vi "HEC28_PEMFC_UserInterface-Testing.vi"() -> ()   [LabVIEW 2020]
uses:
  <vilib>/MakerHub/LINX/Public/Peripherals/Digital/Digital Write 1 Chan.vi
  <vilib>/MakerHub/LINX/Public/Peripherals/Digital/Digital Write N Chans.vi
  <vilib>/MakerHub/LINX/Private/Local IO/LinxDigitalWrite.vi
  <vilib>/MakerHub/LINX/Public/Utilities/Check Channel.vi
  <vilib>/MakerHub/LINX/Public/Utilities/Open Serial.vi
  <instrlib>/NI RMX-400x Loads/Public/Data/Fetch All Measurements (Current).vi
  <instrlib>/NI RMX-400x Loads/Public/Data/Fetch All Measurements (Power).vi
  <instrlib>/NI RMX-400x Loads/Public/Data/Fetch All Measurements (Voltage).vi
  <vilib>/MakerHub/LINX/Private/Utilties/Generate Error.vi
  <vilib>/MakerHub/LINX/LMH-LINX.lvlib
  <instrlib>/NI RMX-400x Loads/NI RMX-400x Loads.lvlib
panel:
  in  "Set Purge Time":dbl=30.0 format="%#_13g"
  in  "Flowrate(SLPM)":dbl=1.5
  out "Power Waveform":dbl[][](graph)
  out "Voltage Waveform":dbl[][](graph)
  out "Hydrogen Pressure":dynamicdata(graph)
  out "Stack Temperatrue":dynamicdata(graph)
  out "Hydrogen Flowrate":dynamicdata(graph)
  out "Filename Out":path
  in  "Filename":path=path "C:/Users/rmah/Desktop/HEC-28-Fuelcell.lvm"
  in  "Enable":bool
  out "Saving Data":bool
  in  "Set Purge Interval (s)":dbl=31.0
  out "Purge Timer (s)":i32
  out "Purge Valve Switch":bool=TRUE
  in  "Set Stack Temp (C)":dbl=20.0 format="%#_13g"
  in  "Channel Mode":i32(ring)=9 items=["CPL"=8, "CPH"=9]
  in  "Power A Value":dbl=10.0
  in  "Power B Value":dbl=5.0
  in  "Power Range":i32(ring)=1 items=["Low", "High", "Medium"]
  in  "Active Power Value":i32(ring) items=["A Value", "B Value"]
  in  "Current Limit":dbl=1.0
  in  "Load COM Port":refnum<visa-resource-name>
  out "Voltage (V)":dbl[](array[numeric])
  out "Power (W)":dbl[](array[numeric])
  out "Current (A)":dbl[](array[numeric])
  out "?":bool=TRUE
  in  "?":bool
  out "?":bool=TRUE
  out "Flowrate (SLPM)":dbl
  out "Temperature (C)":dbl
  in  "LED Switch":bool
  out "Loop Rate (Hz)":u32
  out "Pressure (PSI)":dbl
  # "HEC 28  - FUEL CELL CONTROLLER INTERFACE"
  # "LED Indicator"
  # "Blower Fan"
  # "Hydrogen Supply"
  # "Purge Valve"
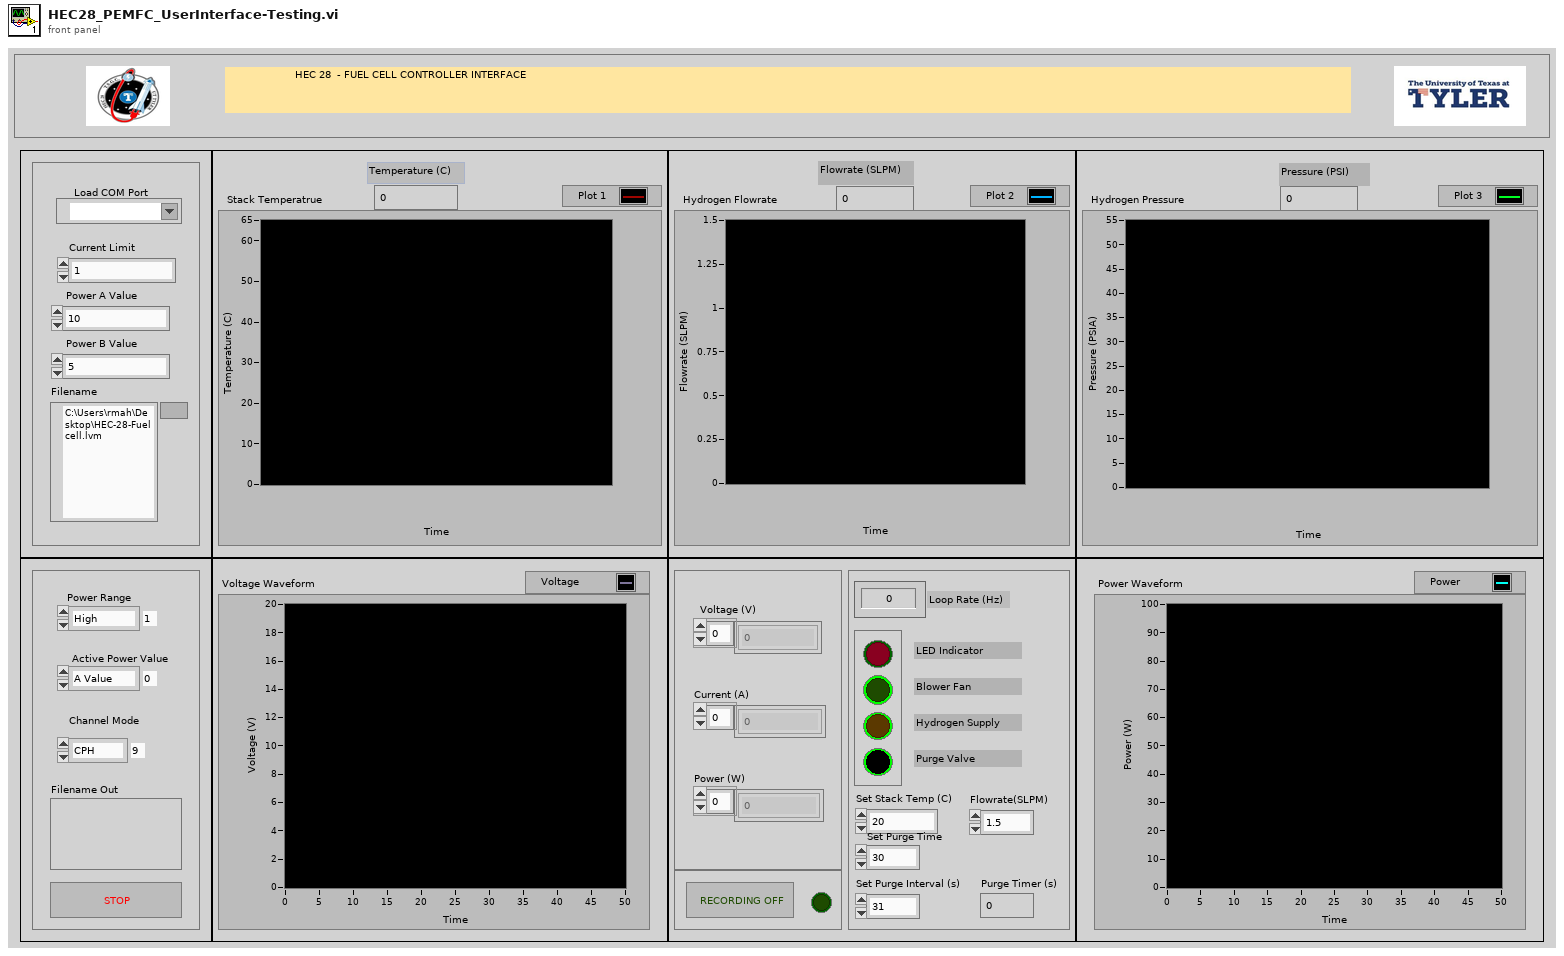
[diagram p1: front panel]
types:
  T1 = typedef "LMH-LINX.lvlib/LINX Ref.ctl" = cluster{"IO":T2, "Interface":T3, "LINX Device Config":T4}
  T2 = typedef "LMH-LINX.lvlib/Platform.ctl" = enum16{"Remote", "Local"}
  T3 = typedef "LMH-LINX.lvlib/Interface.ctl" = enum16{"Serial", "TCP"}
  T4 = typedef "LMH-LINX.lvlib/Device.lvlib/LINX Device Config.ctl" = cluster{"Interface":T3, "COM Port":refnum<visa-resource-name>, "TCP Configuration":T5, "Device Family":u8, "Device ID":u8, "Device Name":string, "TCP Ref":refnum<k5>, "Channels":T6}
  T5 = typedef "LMH-LINX.lvlib/Device.lvlib/TCP Config.ctl" = cluster{"IP Address":string, "Port":u16}
  T6 = typedef "LMH-LINX.lvlib/Channels.ctl" = cluster{"DI":u8[], "DO":u8[], "AI":u8[], "AO":u8[], "PWM":u8[], "QE":u8[], "UART":u8[], "I2C 2":u8[], "SPI":u8[], "CAN":u8[], "Servo":u8[], "AI Ref (V)":dbl, "AI Resolution (Bits)":u8, "AO Ref (V)":dbl, "AO Resolution (Bits)":u8}
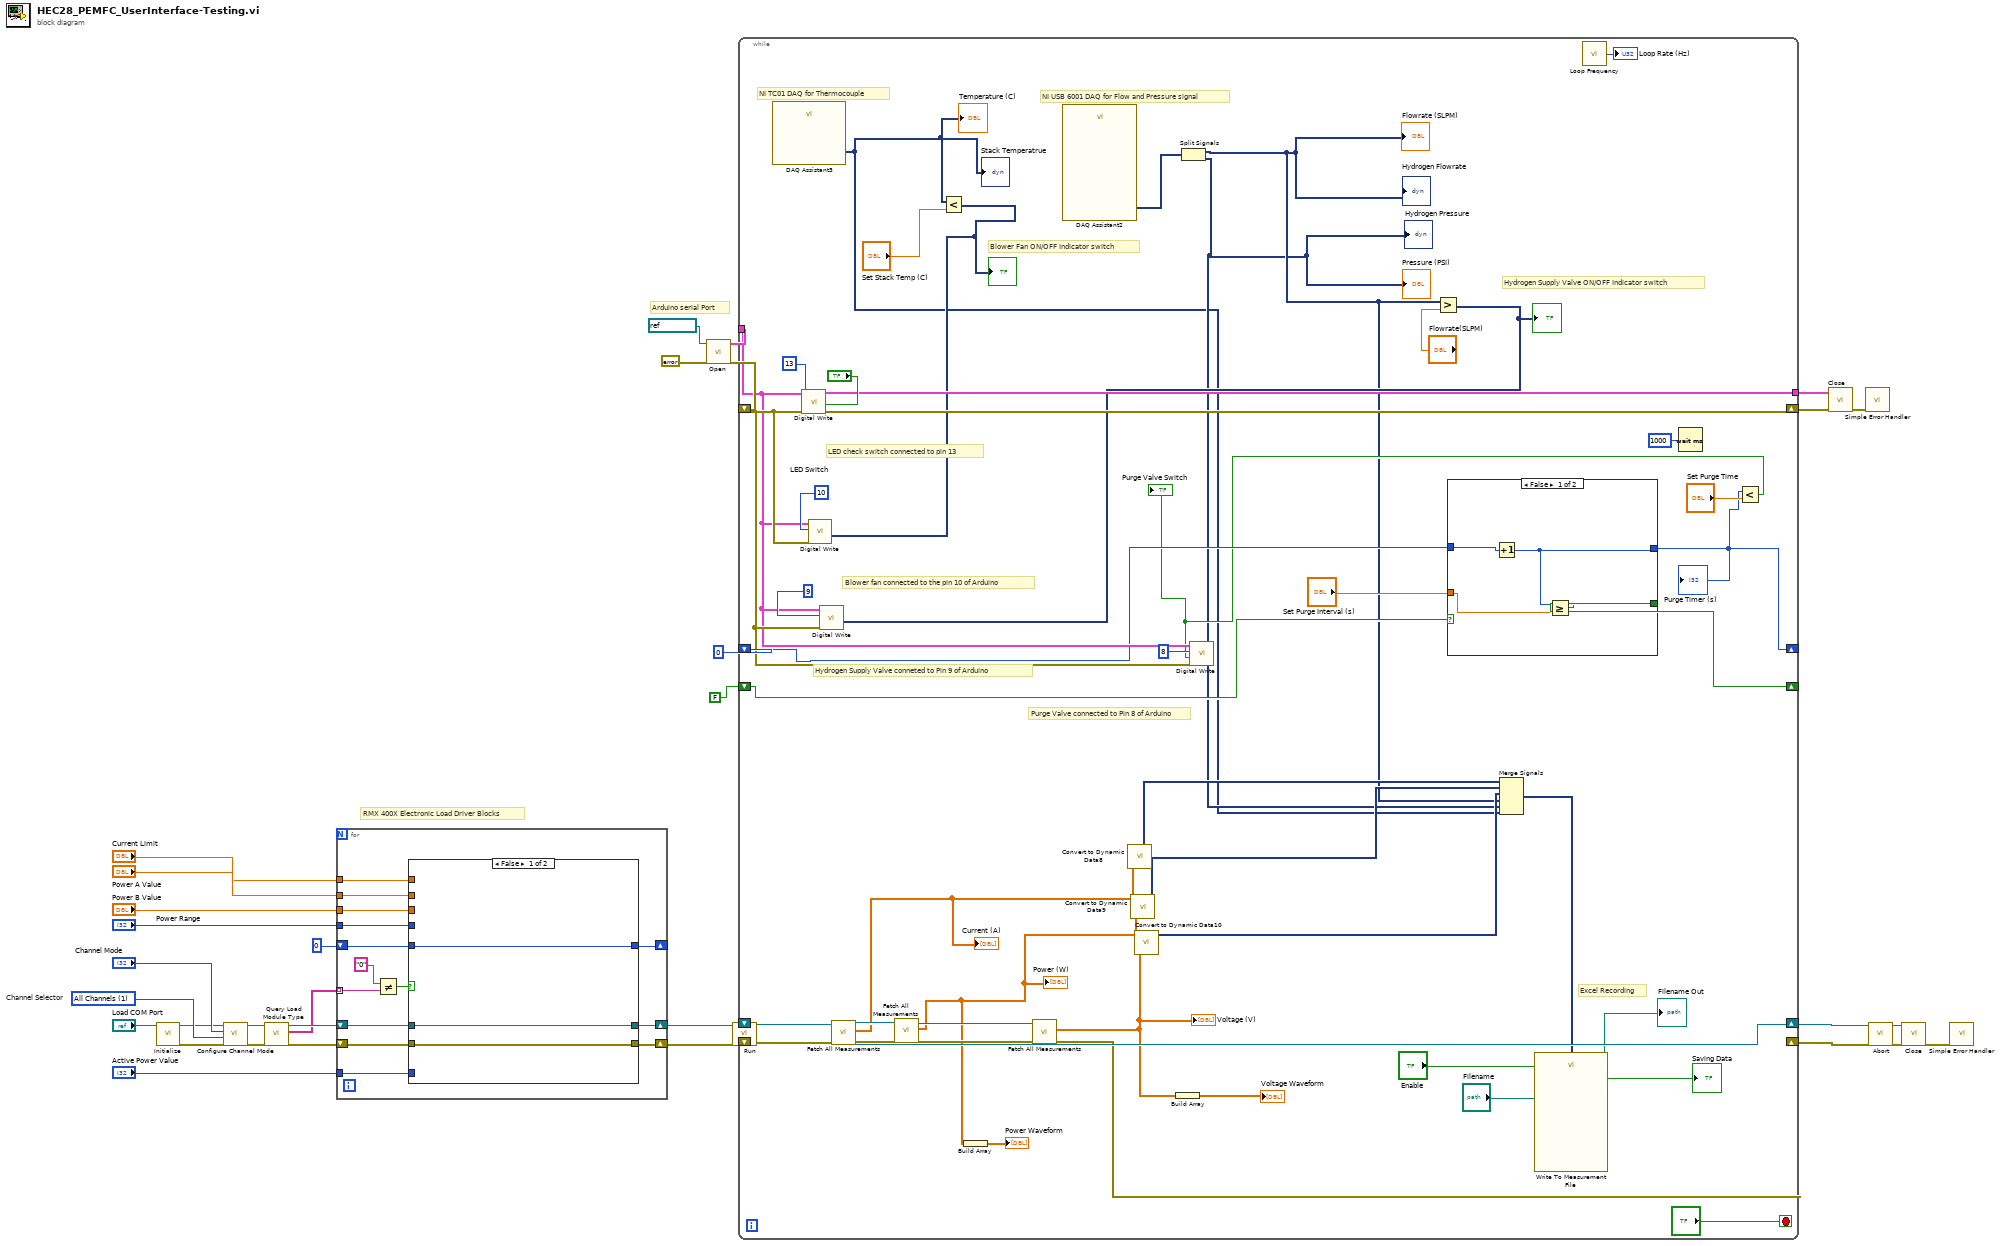
[diagram p0: block diagram]
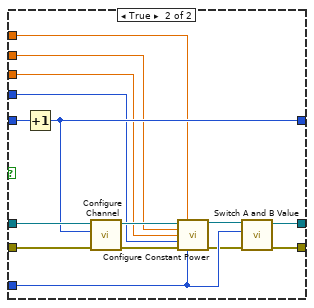
[diagram p2: hidden frame]
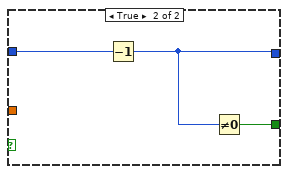
[diagram p3: hidden frame]
diagram:
  w19 = 1 items=["Currently Active Channel", "All Channels"]  # Channel Selector
  # "RMX 400X Electronic Load Driver Blocks"
  # "Arduino serial Port"
  n1 = call <instrlib>:"Initialize.vi"("VISA resource name"="Load COM Port") -> ("error out"=w16:errorcluster, "VISA resource name out"=w15:refnum<visa-resource-name>)  [unwired: 9 in]
  n2 = call <instrlib>:"Configure Channel Mode.vi"("error in (no error)"=w16, "Channel Selector (0: Currently Active Channel)"=w19, "Channel Mode (0: CCL)"="Channel Mode", "VISA resource name"=w15) -> ("error out"=w18:errorcluster, "VISA resource name out"=w17:refnum<visa-resource-name>)  [unwired: 6 in]
  n3 = call <instrlib>:"Query Load Module Type.vi"("error in (no error)"=w18, "VISA resource name"=w17) -> ("error out"=w13:errorcluster, "Load Module Type"=w11:string[], "VISA resource name out"=w12:refnum<visa-resource-name>)  [unwired: 7 in]
  n4 = for {
    tunnel: w11 -> [w48] mode=indexing
    shift-right: [w42] -> _
    shift-left: 0 -> [w43]
    shift-right: [w41] -> w24
    shift-left: w12 -> [w45]
    shift-right: [w40] -> w25
    shift-left: w13 -> [w44]
    tunnel: "Current Limit" -> [w39]
    tunnel: "Power A Value" -> [w38]
    tunnel: "Power B Value" -> [w37]
    tunnel: "Power Range" -> [w36]
    tunnel: "Active Power Value" -> [w35]
    n5 = Not Equal?(x="0", y=w48) -> (x != y?=w46:bool)
    n6 = case shown="False" w46 {
      tunnel: w45 -> [w50 w65]
      tunnel: w44 -> [w49 w64]
      tunnel: w43 -> [w51 w66]
      tunnel: [w51 w63] -> w42
      tunnel: [w50 w54] -> w41
      tunnel: [w49 w56] -> w40
      tunnel: w39 -> [_ w57]
      tunnel: w38 -> [_ w58]
      tunnel: w37 -> [_ w59]
      tunnel: w36 -> [_ w60]
      tunnel: w35 -> [_ w53]
      frame False {
      }
      frame True {
        n7 = Increment(x=w66) -> (x+1=w63:i32)
        n8 = call <instrlib>:"Configure Channel.vi"("error in (no error)"=w64, "Channel (1: Channel 1)"=w63, "VISA resource name"=w65) -> ("error out"=w61:errorcluster, "VISA resource name out"=w62:refnum<visa-resource-name>)  [unwired: 7 in]
        n9 = call <instrlib>:"Configure Constant Power.vi"("VISA resource name"=w62, "Current Limit (20 A)"=w57, "Power A Value (1 W)"=w58, "Power B Value (1 W)"=w59, "Power Range (1: High)"=w60, "error in (no error)"=w61, "Active Power Value (0: A Value)"=w53) -> ("VISA resource name out"=w55:refnum<visa-resource-name>, "error out"=w52:errorcluster)  [unwired: 7 in]
        n10 = call <instrlib>:"Switch A and B Value.vi"("error in (no error)"=w52, "Active Value(0: A Value)"=w53, "VISA resource name"=w55) -> ("error out"=w56:errorcluster, "VISA resource name out"=w54:refnum<visa-resource-name>)  [unwired: 7 in]
      }
    }
  }
  n11 = call-poly <vilib>:"Open.vi"("Error In"=errorcluster {"status"=FALSE, "code"=0, "source"=""}, "Serial Port"=refnum<visa-resource-name> "COM5") -> ("Error Out"=w33:errorcluster, "LINX Resource"=w34:T1)  [unwired: 7 in, 1 out]
  n12 = call <instrlib>:"Run.vi"("error in (no error)"=w25, "VISA resource name"=w24) -> ("error out"=w8:errorcluster, "VISA resource name out"=w9:refnum<visa-resource-name>)  [unwired: 8 in]
  n13 = while {
    tunnel: w34 -> [w95]
    shift-right: [w106] -> w32
    shift-left: w33 -> [w96]
    tunnel: [w107] -> w29
    shift-right: [w98] -> w4
    shift-left: w9 -> [w101]
    shift-right: [w97] -> w3
    shift-left: w8 -> [w100]
    shift-right: [w87] -> _
    shift-left: 0 -> [w90]
    shift-right: [w88] -> _
    shift-left: FALSE -> [w89]
    stop <- "?" stop-if-true
    # "Excel Recording"
    # "Hydrogen Supply Valve ON/OFF Indicator switch"
    # "Blower Fan ON/OFF Indicator switch"
    # "NI TC01 DAQ for Thermocouple"
    # "NI USB 6001 DAQ for Flow and Pressure signal"
    # "LED check switch connected to pin 13"
    # "Blower fan connected to the pin 10 of Arduino"
    # "Hydrogen Supply Valve conneted to Pin 9 of Arduino"
    # "Purge Valve connected to Pin 8 of Arduino"
    n14 = call "DAQ Assistant3"() -> ("data"=w73:dynamicdata)  [unwired: 17 in, 2 out]
    "Temperature (C)" <- w73
    "Stack Temperatrue" <- w73
    n15 = call-poly <vilib>:"Digital Write.vi"("Error In"=w96, "Output Value"="LED Switch", "DO Channel"=u8 13, "LINX Resource"=w95) -> ("Error Out"=w106:errorcluster, "LINX Resource"=w107:T1)  [unwired: 6 in]
    n16 = call-poly <instrlib>:"Fetch All Measurements.vi"("error in (no error)"=w100, "VISA resource name"=w101) -> ("error out"=w104:errorcluster, "Current (A)"=w71:dbl[], "VISA resource name out"=w105:refnum<visa-resource-name>)  [unwired: 7 in]
    "Current (A)" <- w71
    n17 = call-poly <instrlib>:"Fetch All Measurements.vi"("error in (no error)"=w104, "VISA resource name"=w105) -> ("error out"=w102:errorcluster, "Power (W)"=w69:dbl[], "VISA resource name out"=w103:refnum<visa-resource-name>)  [unwired: 7 in]
    "Power (W)" <- w69
    n18 = Less?(x=w73, y="Set Stack Temp (C)") -> (x < y?=w84:dynamicdata)
    "?" <- w84
    n19 = call-poly <vilib>:"Digital Write.vi"("Error In"=w96, "Output Value"=w84, "DO Channel"=u8 10, "LINX Resource"=w95) -> ()  [unwired: 6 in, 2 out]
    n20 = Build Array(w69) -> (→"Power Waveform":dbl[][])
    n21 = call-poly <instrlib>:"Fetch All Measurements.vi"("error in (no error)"=w102, "VISA resource name"=w103) -> ("error out"=w97:errorcluster, "Voltage (V)"=w70:dbl[], "VISA resource name out"=w98:refnum<visa-resource-name>)  [unwired: 7 in]
    "Voltage (V)" <- w70
    n22 = call "DAQ Assistant2"() -> ("data"=w85:dynamicdata)  [unwired: 17 in, 2 out]
    n23 = call "Convert to Dynamic Data8"("Array"=w71) -> ("Dynamic Data Type"=w79:dynamicdata)  [unwired: 3 in]
    n24 = call "Convert to Dynamic Data9"("Array"=w69) -> ("Dynamic Data Type"=w78:dynamicdata)  [unwired: 3 in]
    n25 = call "Convert to Dynamic Data10"("Array"=w70) -> ("Dynamic Data Type"=w77:dynamicdata)  [unwired: 3 in]
    n26 = Build Array(w70) -> (→"Voltage Waveform":dbl[][])
    n27 = Split Signals(w85) -> (w75:dynamicdata, w74:dynamicdata)  [unwired: 2 in]
    "Pressure (PSI)" <- w74
    "Flowrate (SLPM)" <- w75
    "Hydrogen Flowrate" <- w75
    "Hydrogen Pressure" <- w74
    n28 = Greater?(x=w75, y="Flowrate(SLPM)") -> (0:w99:dynamicdata)
    "?" <- w99
    n29 = call-poly <vilib>:"Digital Write.vi"("Error In"=w96, "Output Value"=w99, "DO Channel"=u8 9, "LINX Resource"=w95) -> ()  [unwired: 6 in, 2 out]
    n30 = case shown="False" w89 {
      tunnel: w90 -> [w118 w121]
      tunnel: [w117 w120] -> w87
      tunnel: [w115 w119] -> w88
      tunnel: "Set Purge Interval (s)" -> [w116 _]
      frame False {
        n31 = Increment(x=w118) -> (x+1=w117:i32)
        n32 = Greater Or Equal?(x=w117, y=w116) -> (x >= y?=w115:bool)
      }
      frame True {
        n33 = Decrement(x=w121) -> (x-1=w120:i32)
        n34 = Not Equal To 0?(x=w120) -> (x != 0?=w119:bool)
      }
    }
    "Purge Timer (s)" <- w87
    n35 = Merge Signals(w79, w78, w77, w75, w74, w73) -> (w83:dynamicdata)
    n36 = call "Write To Measurement File"("Signals"=w83, "Enable"="Enable", "Filename"="Filename") -> ("Filename Out"=→"Filename Out":path, "Saving Data"=→"Saving Data":bool)  [unwired: 14 in, 1 out]
    n37 = call <vilib>:"Loop Frequency.vi"() -> ("Loop Rate (Hz)"=→"Loop Rate (Hz)":u32)
    n38 = Wait (ms)(milliseconds to wait=u32 1000) -> ()  [unwired: 1 out]
    n39 = Less?(x=w87, y="Set Purge Time") -> (x < y?=w86:bool)
    "Purge Valve Switch" <- w86
    n40 = call-poly <vilib>:"Digital Write.vi"("Error In"=w96, "Output Value"=w86, "DO Channel"=u8 8, "LINX Resource"=w95) -> ()  [unwired: 6 in, 2 out]
  }
  n41 = call <vilib>:"Close.vi"("Error In"=w32, "LINX Resource"=w29) -> ("Error Out"=w31:errorcluster)  [unwired: 9 in]
  n42 = call <vilib>:"Simple Error Handler.vi"("error in (no error)"=w31) -> ()  [unwired: 4 in, 5 out]
  n43 = call <instrlib>:"Abort.vi"("error in (no error)"=w3, "VISA resource name"=w4) -> ("error out"=w7:errorcluster, "VISA resource name out"=w6:refnum<visa-resource-name>)  [unwired: 8 in]
  n44 = call <vilib>:"Close.vi"("error in (no error)"=w7, "VISA resource name"=w6) -> ("error out"=w5:errorcluster)  [unwired: 9 in]
  n45 = call <vilib>:"Simple Error Handler.vi"("error in (no error)"=w5) -> ()  [unwired: 4 in, 5 out]
